vi "Move.vi"(8 "error in (no error)":errorcluster, 10 "Position":cluster{"x":dbl, "y":dbl, "z":dbl}, 11 "Gantry Class in":refnum<class "Gantry Class.lvclass">) -> (0 "error out":errorcluster, 3 "Gantry Class out":refnum<class "Gantry Class.lvclass">)   [LabVIEW 2011, in "Gantry Class.lvclass"]
uses:
  Gantry Class.lvclass
  Gantry Class.lvclass/Gantry Class.ctl
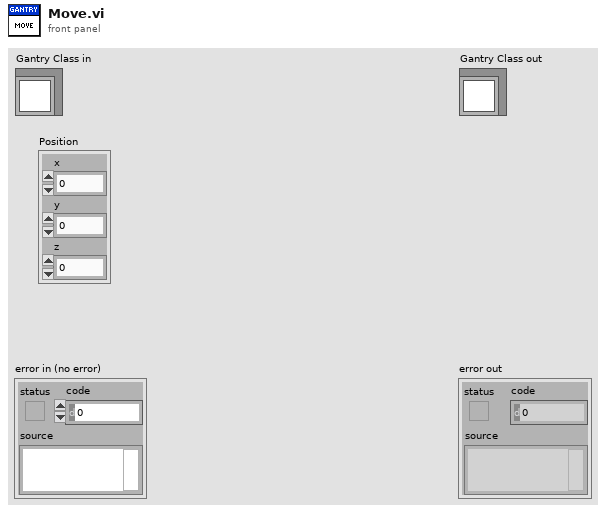
[diagram p1: front panel]
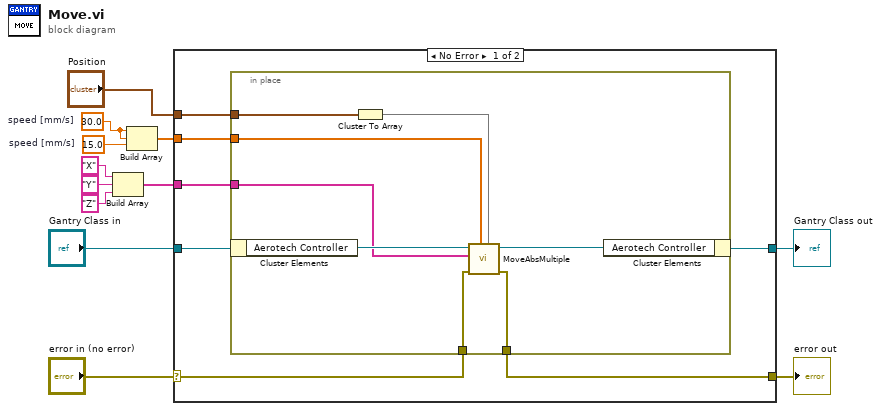
[diagram p0: block diagram]
diagram:
  w3 = 15.0  # speed [mm/s]
  w4 = 30.0  # speed [mm/s]
  n1 = Build Array("X", "Y", "Z") -> (w5:string[])
  n2 = Build Array(w4, w4, w3) -> (w2:dbl[])
  n3 = case shown="No Error" "error in (no error)" {
    selector: "error in (no error)" -> [w17 w29]
    tunnel: [w16 w29] -> w11
    tunnel: [w18 w28] -> w9
    tunnel: "Gantry Class in" -> [w19 w28]
    tunnel: w5 -> [w15 _]
    tunnel: w2 -> [w14 _]
    tunnel: "Position" -> [w13 _]
    frame No Error {
      n4 = in-place {
        in-place-border: w17 -> [w25]
        in-place-border: [w24] -> w16
        in-place-border: w15 -> [w23]
        in-place-border: w14 -> [w21]
        in-place-border: w13 -> [w22]
        n5 = in-place-cluster #1(w19) -> ("Aerotech Controller"=w27:refnum<k24>)
        n6 = Cluster To Array(cluster=w22) -> (array=w20:dbl[])
        n7 = call <userlib>:"MoveAbsMultiple.vi"("positions"=w20, "speeds"=w21, "error in (no error)"=w25, "axis names"=w23, "controller in"=w27) -> ("error out"=w24:errorcluster, "controller out"=w26:refnum<k24>)  [unwired: 5 in]
        n8 = in-place-cluster #1("Aerotech Controller"=w26) -> (w18:refnum<class "Gantry Class.lvclass">)
      }
    }
    frame Error {
    }
  }
  "error out" <- w11
  "Gantry Class out" <- w9
